vi "LiftQuadratic.vi"(7 "Original Position":dbl, 10 "Current Position":dbl, 11 "Setpoint":dbl) -> (2 "Output":dbl)   [LabVIEW 2017]
panel:
  in  "Scale":dbl=1.2
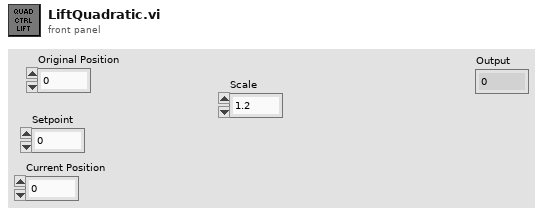
[diagram p1: front panel]
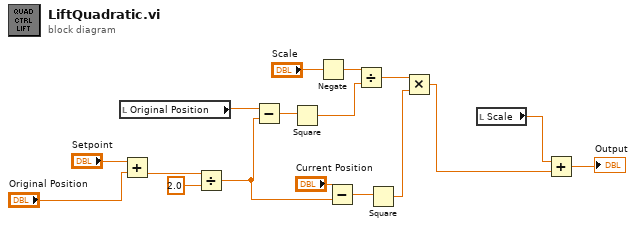
[diagram p0: block diagram]
diagram:
  n1 = local read "Original Position"() -> (w11:dbl)
  n2 = Add(x="Setpoint", y="Original Position") -> (x+y=w13:dbl)
  n3 = Divide(x=w13, y=2.0) -> (x/y=w4:dbl)
  n4 = Subtract(x=w11, y=w4) -> (x-y=w10:dbl)
  n5 = Square(x=w10) -> (x^2=w7:dbl)
  n6 = Negate(x="Scale") -> (-x=w8:dbl)
  n7 = Subtract(x="Current Position", y=w4) -> (x-y=w3:dbl)
  n8 = Divide(x=w8, y=w7) -> (x/y=w6:dbl)
  n9 = Square(x=w3) -> (x^2=w2:dbl)
  n10 = Multiply(x=w6, y=w2) -> (x*y=w1:dbl)
  n11 = local read "Scale"() -> (w16:dbl)
  n12 = Add(x=w16, y=w1) -> (x+y=→"Output":dbl)
